vi "Get_DAQmxTask.vi"(8 "error in (no error)":errorcluster, 10 "Task name":string, 11 "DAQmxTaksContainer_General in":refnum<class "DAQmxTaksContainer_General.lvclass">) -> (0 "error out":errorcluster, 2 "DAQmx Task":refnum<class "DAQmxTask.lvclass">, 3 "DAQmxTaksContainer_General out":refnum<class "DAQmxTaksContainer_General.lvclass">)   [LabVIEW 2020, in "DAQmxTaksContainer_General.lvclass"]
uses:
  DAQmxTaksContainer_General.lvclass
  DAQmxTask.lvclass
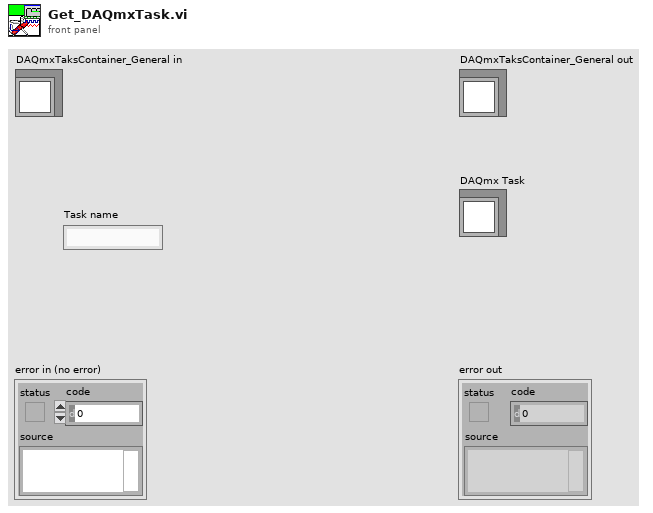
[diagram p1: front panel]
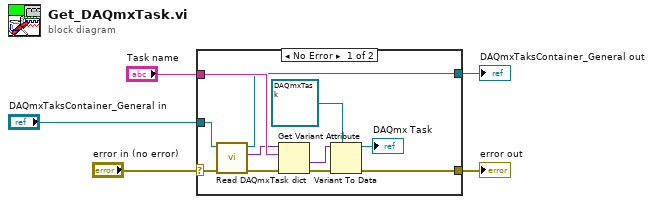
[diagram p0: block diagram]
diagram:
  n1 = case shown="No Error" "error in (no error)" {
    selector: "error in (no error)" -> [w8 w18]
    tunnel: [w13 w18] -> w3
    tunnel: [w6 w17] -> w4
    tunnel: "DAQmxTaksContainer_General in" -> [w10 w17]
    tunnel: "Task name" -> [w16 _]
    frame No Error {
      n2 = call-dynamic "Read DAQmxTask dict.vi"("error in (no error)"=w8, "DAQmxTaskContainer_general in"=w10) -> ("error out"=w7:errorcluster, "DAQmxTask dict"=w9:variant, "DAQmxTaskContainer_general out"=w6:refnum<class "DAQmxTaksContainer_General.lvclass">)  [unwired: 7 in]
      n3 = Get Variant Attribute(Variant=w9, name=w16, error in=w7) -> (value=w15:variant, error out=w14:errorcluster)  [unwired: 1 in, 2 out]
      n4 = Variant To Data(error in=w14, type=refnum<class "DAQmxTask.lvclass"> refnum ("DAQmxTask.lvclass"), Variant=w15) -> (data=→"DAQmx Task":refnum<class "DAQmxTask.lvclass">, error out=w13:errorcluster)
    }
    frame Error {
    }
  }
  "error out" <- w3
  "DAQmxTaksContainer_General out" <- w4
